vi "Get Number of Columns.vi"(6 "wait for reply (T)":bool=TRUE, 8 "error in":errorcluster) -> (0 "error out":errorcluster, 1 "timed out?":bool, 3 "Number Of Columns":i32)   [LabVIEW 2020, in "Manejador archivo.lvlib"]
doc: "_____\nCreated using DQMH Framework: Event Scripter 7.1.0.1490."
uses:
  Manejador archivo.lvlib
  Get Number of Columns Argument--cluster.ctl
  Get Number of Columns (Reply Payload)--cluster.ctl
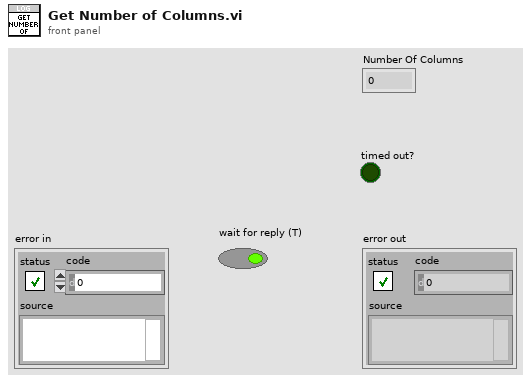
[diagram p1: front panel]
types:
  T1 = typedef "Manejador archivo.lvlib/Get Number of Columns Argument--cluster.ctl" = cluster{"Wait Notifier":refnum<notifier>, "wait for reply":bool}
  T2 = typedef "Manejador archivo.lvlib/Request Events--cluster.ctl" = cluster{"Stop Module":refnum<user-event>, "Show Panel":refnum<user-event>, "Hide Panel":refnum<user-event>, "Get Module Execution Status":refnum<user-event>, "Show Diagram":refnum<user-event>, "Set Column Headers":refnum<user-event>, "View File":refnum<user-event>, "Set File Path":refnum<user-event>, "Set File Settings":refnum<user-event>, "Log Data":refnum<user-event>, "Set File Format":refnum<user-event>, "Close File":refnum<user-event>, "Get Number of Columns":refnum<user-event>}
  T3 = typedef "Manejador archivo.lvlib/Get Number of Columns (Reply Payload)--cluster.ctl" = cluster{"error":errorcluster, "Number Of Columns":i32}
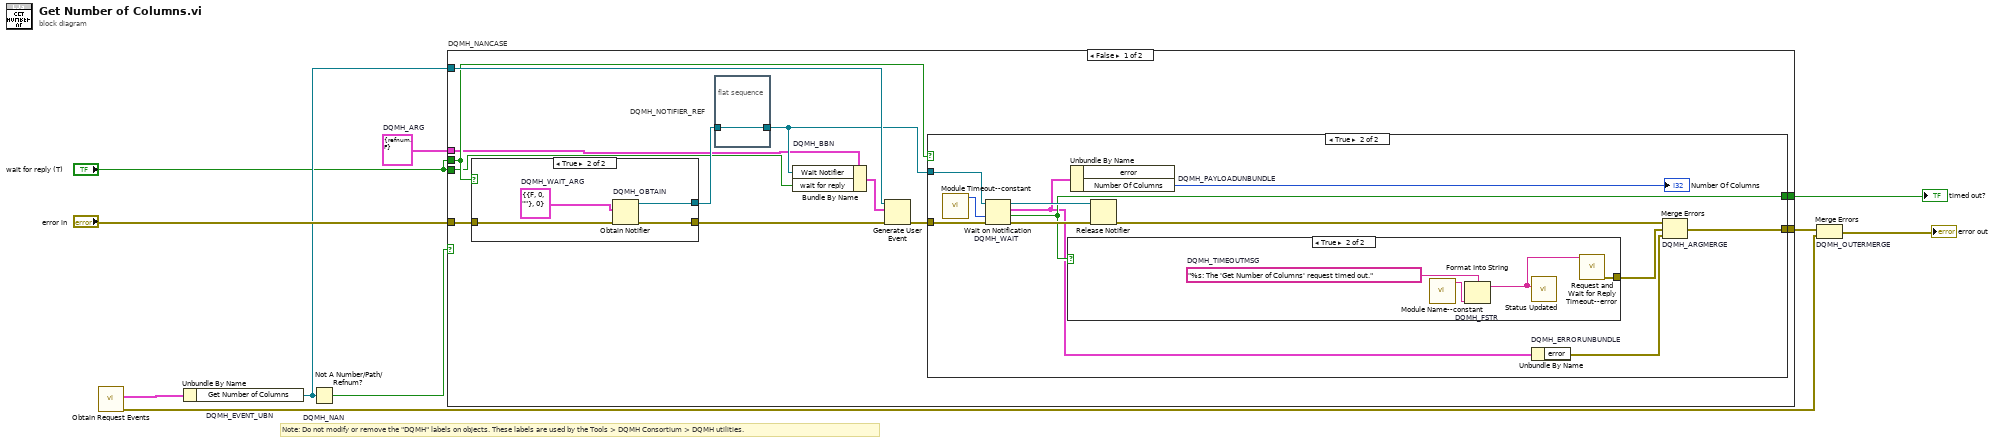
[diagram p0: block diagram]
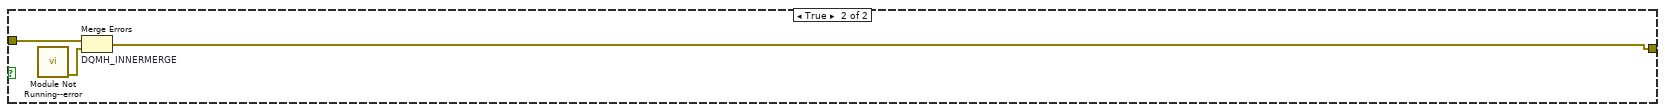
[diagram p5: hidden frame]
diagram:
  w3 = T1 {"Wait Notifier"=refnum, "wait for reply"=FALSE}  # DQMH_ARG
  # "Note: Do not modify or remove the \"DQMH\" labels on objects. These labels are used by the Tools > DQMH Consortium > DQMH utilities."
  n1 = call "Obtain Request Events.vi"() -> ("error out"=w7:errorcluster, "Manejador archivo Request Events"=w1:T2)  [unwired: 10 in]
  n2 = Unbundle By Name "DQMH_EVENT_UBN"(w1) -> ("Get Number of Columns"=w4:refnum<user-event>)
  n3 = Not A Number/Path/Refnum? "DQMH_NAN"(number/path/refnum=w4) -> (NaN/Path/Refnum?=w5:bool)
  n4 = case "DQMH_NANCASE" shown="False" w5 {
    tunnel: "error in" -> [w22 w48]
    tunnel: w4 -> [w18 _]
    tunnel: [w19 w47] -> w8
    tunnel: [w17 _] -> w6
    tunnel: "wait for reply (T)" -> [w15 _]
    tunnel: w3 -> [w12 _]
    tunnel: "wait for reply (T)" -> [w11 _]
    frame False {
      n5 = case shown="True" w15 {
        tunnel: w22 -> [w41 w45]
        tunnel: [w41 w44] -> w20
        tunnel: [_ w42] -> w14
        frame False {
        }
        frame True {
          w43 = T3 {"error"={"status"=FALSE, "code"=0, "source"=""}, "Number Of Columns"=0}  # DQMH_WAIT_ARG
          n6 = Obtain Notifier "DQMH_OBTAIN"(notification data type=w43, error in (no error)=w45) -> (notifier out=w42:refnum<notifier>, error out=w44:errorcluster)  [unwired: 2 in, 1 out]
        }
      }
      n7 = flat-sequence "DQMH_NOTIFIER_REF" {
        tunnel: w14 -> [w23]
        tunnel: [w23] -> w13
        frame #0 {
        }
      }
      n8 = Bundle By Name "DQMH_BBN"(cluster=w12, "Wait Notifier"=w13, "wait for reply"=w11) -> (w16:T1)
      n9 = Generate User Event(user event=w18, event data cluster=w16, error in=w20) -> (error out=w21:errorcluster)  [unwired: 1 in, 1 out]
      n10 = case shown="True" w15 {
        tunnel: w21 -> [w24 w36]
        tunnel: w13 -> [_ w30]
        tunnel: [_ w28] -> w17
        tunnel: [w24 w35] -> w19
        frame False {
        }
        frame True {
          n11 = call "Module Timeout--constant.vi"() -> ("Module Timeout"=w26:i32)  [unwired: 11 in]
          n12 = Wait on Notification "DQMH_WAIT"(notifier=w30, timeout in ms (-1)=w26, error in (no error)=w36) -> (notifier out=w29:refnum<notifier>, notification=w27:T3, timed out?=w28:bool, error out=w34:errorcluster)  [unwired: 1 in]
          n13 = case shown="True" w28 {
            tunnel: [_ w40] -> w31
            frame False {
            }
            frame True {
              w39 = "%s: The 'Get Number of Columns' request timed out."  # DQMH_TIMEOUTMSG
              n14 = call "Module Name--constant.vi"() -> ("Module Name"=w37:string)  [unwired: 11 in]
              n15 = Format Into String "DQMH_FSTR"(format string=w39, w37) -> (resulting string=w38:string)  [unwired: 2 in, 1 out]
              n16 = call "Status Updated.vi"("Status"=w38) -> ()  [unwired: 10 in, 1 out]
              n17 = call "Request and Wait for Reply Timeout--error.vi"("Error Message"=w38) -> ("error out"=w40:errorcluster)  [unwired: 10 in]
            }
          }
          n18 = Unbundle By Name "DQMH_PAYLOADUNBUNDLE"(w27) -> ("Number Of Columns"=→"Number Of Columns":i32)  [unwired: 1 out]
          n19 = Release Notifier(notifier=w29, error in (no error)=w34) -> (error out=w33:errorcluster)  [unwired: 1 in, 2 out]
          n20 = Unbundle By Name "DQMH_ERRORUNBUNDLE"(w27) -> ("error"=w32:errorcluster)
          n21 = Merge Errors "DQMH_ARGMERGE"(w33, w31, w32) -> (w35:errorcluster)
        }
      }
    }
    frame True {
      n22 = call "Module Not Running--error.vi"() -> ("error out"=w46:errorcluster)  [unwired: 11 in]
      n23 = Merge Errors "DQMH_INNERMERGE"(w48, w46) -> (w47:errorcluster)
    }
  }
  "timed out?" <- w6
  n24 = Merge Errors "DQMH_OUTERMERGE"(w8, w7) -> (→"error out":errorcluster)
